vi "Init Module.vi"(8 "error in (no error)":errorcluster, 10 "Close Master Reference (F)":bool, 11 "Cloneable Module Admin in":refnum<class "Delacor_lib_QMH_Cloneable Module Admin.lvclass">) -> (0 "error out":errorcluster, 2 "Thermal Chamber Request Events":T1, 3 "Cloneable Module Admin out":refnum<class "Delacor_lib_QMH_Cloneable Module Admin.lvclass">)   [LabVIEW 2024, in "Thermal Chamber.lvlib"]
doc: "Initialize the module by creating Broadcast Events, Request Events, and synchronization rendezvous. Also, since this is a cloneable module, add it to the cloneable registry and update the Module Admin class.\n\nSee the block diagram for an explanation of the 'Close Master Reference' parameter.\n_____\nBased on DQMH Project Template 6.0.0.91.\n\n<b>Note:</b> This VI was modified by the <b>Validate DQMH Module</b> tool to add the 'Show Main VI Diagram on Init' functionality included in DQMH 6.1."
uses:
  Thermal Chamber.lvlib
  <vilib>/Delacor/Delacor QMH/Libraries/Cloneable Module Admin_class/Delacor_lib_QMH_Cloneable Module Admin.lvclass
  C:/Program Files/National Instruments/LabVIEW 2024/vi.lib/Delacor/Delacor QMH/Libraries/Module Admin_class/Delacor_lib_QMH_Module Admin.lvclass
  Request Events--cluster.ctl
  Stop Argument--cluster.ctl
  Show Panel Argument--cluster.ctl
  Hide Panel Argument--cluster.ctl
  Show Diagram Argument--cluster.ctl
  Get Module Execution Status Argument--cluster.ctl
  Initialize Argument--cluster.ctl
  Class Libraries/Process Controller/Controls/Class Selector--Enum.ctl
  Initialize (Reply Payload)--cluster.ctl
  Shutdown Argument--cluster.ctl
  Shutdown (Reply Payload)--cluster.ctl
  Set Temp Setpoint Argument--cluster.ctl
  Class Libraries/Process Controller/Controls/Temp Data--Cluster.ctl
  Class Libraries/Process Controller/Controls/Temperature Units--Enum.ctl
  Set Temp Setpoint (Reply Payload)--cluster.ctl
  Set Temp Ramp Rate Argument--cluster.ctl
  Class Libraries/Process Controller/Controls/Temp Ramp Rate Data--Cluster.ctl
  Class Libraries/Process Controller/Controls/Rate Units--Enum.ctl
  Set Temp Ramp Rate (Reply Payload)--cluster.ctl
  Set Temp Control State Argument--cluster.ctl
  Set Temp Control State (Reply Payload)--cluster.ctl
  Get Temp Feedback Argument--cluster.ctl
  Get Temp Feedback (Reply Payload)--cluster.ctl
  Read Controller Data Argument--cluster.ctl
  Read Controller Data (Reply Payload)--cluster.ctl
  <vilib>/Delacor/Delacor QMH/Libraries/Module Admin_class/Delacor_lib_QMH_Module Admin.lvclass/Delacor_lib_QMH_Module Admin.ctl
  <vilib>/Delacor/Delacor QMH/Libraries/Cloneable Module Admin_class/Delacor_lib_QMH_Cloneable Module Admin.lvclass/Delacor_lib_QMH_Cloneable Module Admin.ctl
  <vilib>/Delacor/Delacor QMH/Libraries/Module Admin_class/Delacor_lib_QMH_Get External Launch.vi
  <vilib>/Delacor/Delacor QMH/Libraries/Cloneable Module Admin_class/Delacor_lib_QMH_Get Module ID.vi
  <vilib>/Delacor/Delacor QMH/Libraries/Cloneable Module Admin_class/Delacor_lib_QMH_Set Close Master Reference.vi
  <vilib>/Delacor/Delacor QMH/Libraries/Cloneable Module Admin_class/Delacor_lib_QMH_Set First.vi
  Clone Registration/Clone Registration.lvlib
  Class Libraries/Process Controller/_Thermal Process Controller.lvclass
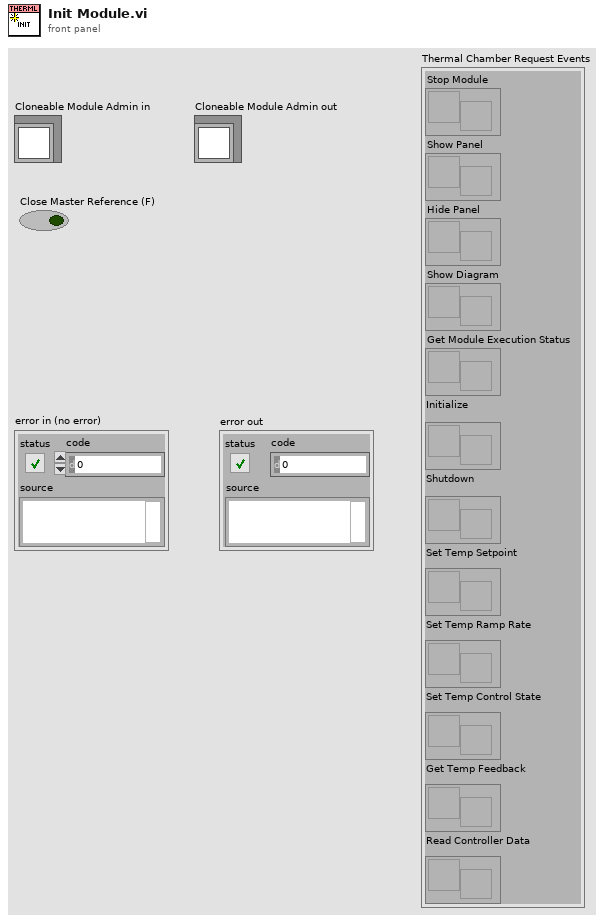
[diagram p1: front panel]
types:
  T1 = typedef "Thermal Chamber.lvlib/Request Events--cluster.ctl" = cluster{"Stop Module":refnum<user-event>, "Show Panel":refnum<user-event>, "Hide Panel":refnum<user-event>, "Show Diagram":refnum<user-event>, "Get Module Execution Status":refnum<user-event>, "Initialize":refnum<user-event>, "Shutdown":refnum<user-event>, "Set Temp Setpoint":refnum<user-event>, "Set Temp Ramp Rate":refnum<user-event>, "Set Temp Control State":refnum<user-event>, "Get Temp Feedback":refnum<user-event>, "Read Controller Data":refnum<user-event>}
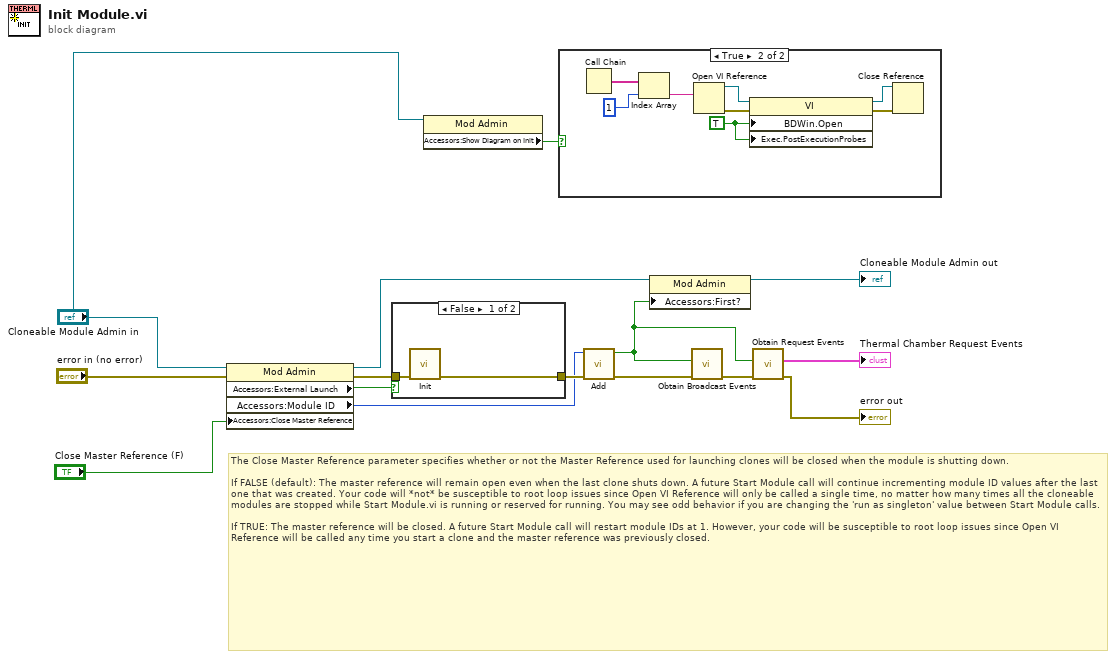
[diagram p0: block diagram]
diagram:
  # "The Close Master Reference parameter specifies whether or not the Master Reference used for launching clones will be closed when the module is shutting down. \n\nIf FALSE (default): The master reference will remain open even when the last clone shuts down. A future Start Module call will continue incrementing module ID values after the last one that was created. Your code will *not* be susceptible to root loop issues since Open VI Reference will only be called a single time, no matter how many times all the cloneable modules are stopped while Start Module.vi is running or reserved for running. You may see odd behavior if you are changing the 'run as singleton' value between Start Module calls.\n\nIf TRUE: The master reference will be closed. A future Start Module call will restart module IDs at 1. However, your code will be susceptible to root loop issues since Open VI Reference will be called any time you start a clone and the master reference was previously closed."
  n1 = property class="Mod Admin"(reference="Cloneable Module Admin in", error in="error in (no error)", "Accessors:Close Master Reference"="Close Master Reference (F)") -> (reference out=w9:refnum<class "Delacor_lib_QMH_Cloneable Module Admin.lvclass">, error out=w4:errorcluster, "Accessors:External Launch"=w8:bool, "Accessors:Module ID"=w3:i32)
  n2 = case "External Launch?" shown="False" w8 {
    tunnel: [w17 w18] -> w14
    tunnel: w4 -> [w16 w18]
    frame False {
      n3 = call "Init.vi"("error in (no error)"=w16) -> ("error out"=w17:errorcluster)  [unwired: 7 in, 3 out]
    }
    frame True {
      # "Init of Clone's registration\nhappened at Start Module.vi"
    }
  }
  n4 = property class="Mod Admin"(reference="Cloneable Module Admin in") -> ("Accessors:Show Diagram on Init"=w1:bool)  [unwired: 1 in, 2 out]
  n5 = case shown="True" w1 {
    frame False {
    }
    frame True {
      w22 = TRUE ("Block Diagram Window:Open")
      n6 = Call Chain() -> (call chain=w26:string[])
      n7 = Index Array(array=w26, index=1) -> (element=w19:string)
      n8 = Open VI Reference(vi path=w19) -> (vi reference=w23:refnum<vi>, error out=w24:errorcluster)  [unwired: 5 in]
      n9 = property class="VI"(reference=w23, error in=w24, "BDWin.Open"=w22, "Exec.PostExecutionProbes"=w22) -> (reference out=w20:refnum<vi>, error out=w21:errorcluster)
      n10 = Close Reference(reference=w20, error in (no error)=w21) -> ()  [unwired: 1 out]
    }
  }
  n11 = call "Add.vi"("error in (no error)"=w14, "Module ID"=w3) -> ("error out"=w15:errorcluster, "First?"=w10:bool)  [unwired: 7 in, 1 out]
  n12 = property class="Mod Admin"(reference=w9, "Accessors:First?"=w10) -> (reference out=→"Cloneable Module Admin out":refnum<class "Delacor_lib_QMH_Cloneable Module Admin.lvclass">)  [unwired: 1 in, 1 out]
  n13 = call "Obtain Broadcast Events.vi"("error in (no error)"=w15, "Create New? (F)"=w10) -> ("error out"=w13:errorcluster)  [unwired: 8 in, 1 out]
  n14 = call "Obtain Request Events.vi"("error in (no error)"=w13, "Create New? (F)"=w10) -> ("error out"=→"error out":errorcluster, "Thermal Chamber Request Events"=→"Thermal Chamber Request Events":T1)  [unwired: 8 in]
